vi "Single Line Digital Counter.vi"(6 "Digital Line - Previous":bool, 7 "Counts per pulse":i32=2, 9 "Digital Line":bool, 11 "Count In":i32) -> (3 "Count Out":i32)   [LabVIEW 2014]
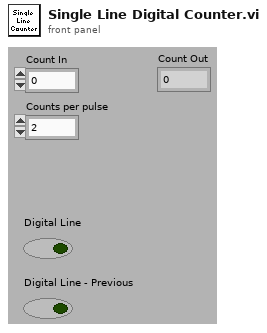
[diagram p1: front panel]
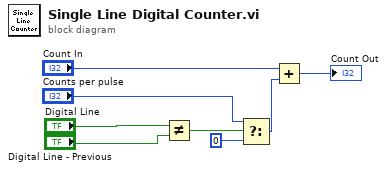
[diagram p0: block diagram]
diagram:
  n1 = Not Equal?(x="Digital Line", y="Digital Line - Previous") -> (x != y?=w6:bool)
  n2 = Select(t="Counts per pulse", s=w6, f=0 ("y")) -> (s? t:f=w1:i32)
  n3 = Add(x="Count In", y=w1) -> (x+y=→"Count Out":i32)
